vi "LaunchICalULInstaller.vi"   [LabVIEW 2009]
uses:
  <vilib>/Utility/sysdir.llb/System Directory Type.ctl
types:
  T1 = typedef "System Directory Type.ctl" = i32
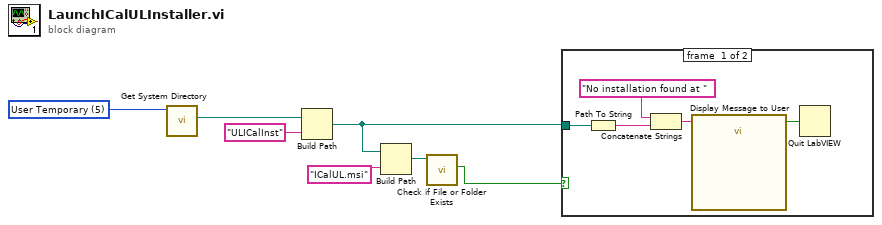
[diagram p0: block diagram]
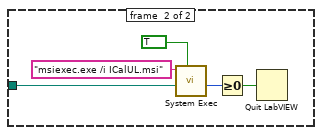
[diagram p2: hidden frame]
diagram:
  w7 = T1 5 items=["User Home", "User Desktop", "User Documents", "User Application Data", "User Preferences", "User Temporary", "Public Documents", "Public Application Data", "Public Preferences", "System Core Libraries", "System Installed Libraries", "Application Files", "Boot Volume Root"] ("system directory type")
  n1 = call <vilib>:"Get System Directory.vi"("system directory type"=w7) -> ("system directory"=w6:path)  [unwired: 10 in]
  n2 = Build Path(base path=w6, name or relative path="ULICalInst") -> (appended path=w1:path)
  n3 = Build Path(base path=w1, name or relative path="ICalUL.msi") -> (appended path=w3:path)
  n4 = call <vilib>:"Check if File or Folder Exists.vi"("path"=w3) -> ("file or folder exists?"=w4:bool)  [unwired: 8 in, 2 out]
  n5 = case shown="False" w4 {
    tunnel: w1 -> [w11 w15]
    frame #0 {
      n6 = Path To String(path=w11) -> (string=w9:string)
      n7 = Concatenate Strings("No installation found at " ("string"), w9) -> (w10:string)
      n8 = call "Display Message to User"("Message"=w10) -> ("OK"=w12:bool)  [unwired: 9 in, 1 out]
      n9 = Quit LabVIEW(quit? (T)=w12) -> ()
    }
    frame #1 {
      n10 = call <vilib>:"System Exec.vi"("wait until completion? (T)"=TRUE, "working directory"=w15, "command line"="msiexec.exe /i ICalUL.msi") -> ("return code"=w13:i32)  [unwired: 5 in, 3 out]
      n11 = Greater Or Equal To 0?(x=w13) -> (x >= 0?=w14:bool)
      n12 = Quit LabVIEW(quit? (T)=w14) -> ()
    }
  }
